vi "test Multi FPGA No Bitfile.vi"(8 "error in (no error)":errorcluster, 11 "TestCase in":refnum<class "Mutation Test Case.lvclass">) -> (0 "error out":errorcluster, 3 "TestCase out":refnum<class "Mutation Test Case.lvclass">)   [LabVIEW 2020, in "Mutation Test Case.lvclass"]
uses:
  Mutation Test Case.lvclass
  Shared/Properties.vi
  <vilib>/NI VeriStand/Custom Device API/Get Item Property (String).vi
  <vilib>/addons/_JKI Toolkits/VI Tester/TestCase.llb/TestCase.lvclass
  System Explorer/Engine Simulation Toolkit System Explorer.lvlib
  <vilib>/NI VeriStand/Custom Device API/Custom Device API.lvlib
  Shared/Engine Simulation Toolkit Shared.lvlib
  C:/Program Files (x86)/National Instruments/LabVIEW 2020/vi.lib/addons/_JKI Toolkits/VI Tester/TestCase.llb/TestCase.lvclass
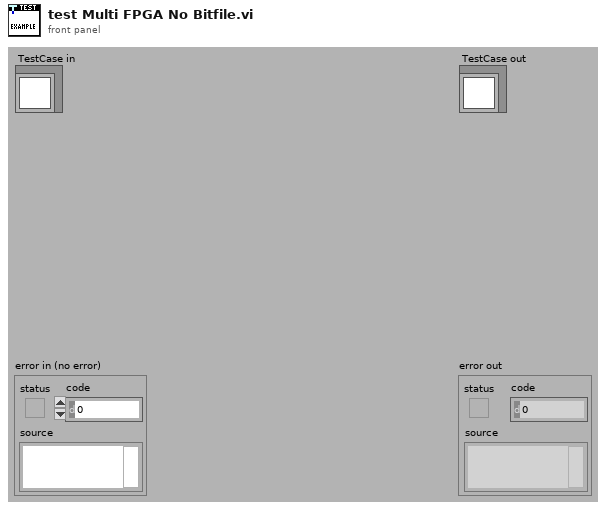
[diagram p1: front panel]
types:
  T1 = typedef "Custom Device API.lvlib/Custom Device Item Ref.ctl" = u64
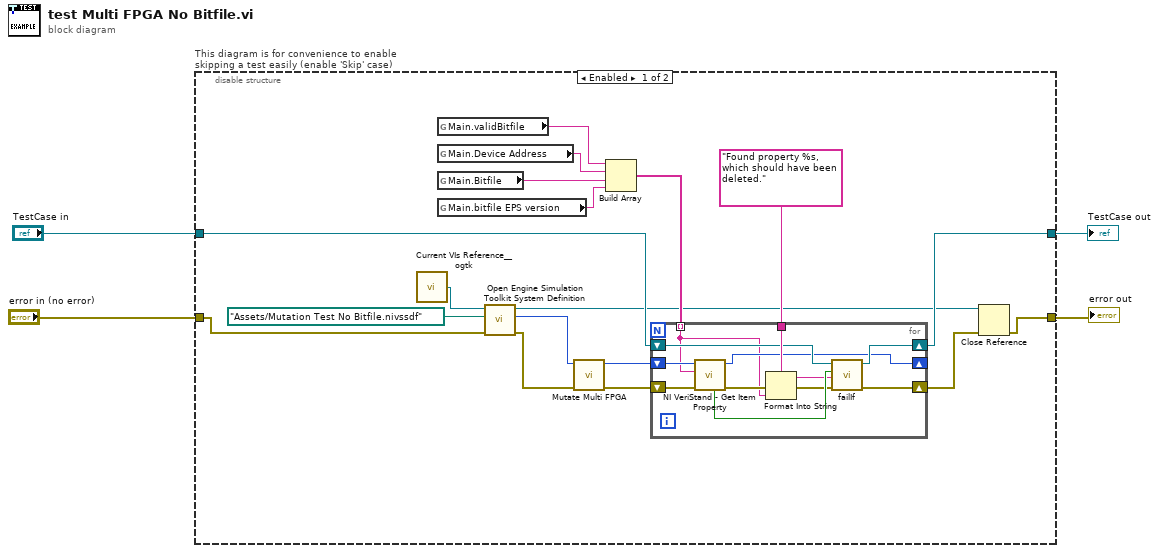
[diagram p0: block diagram]
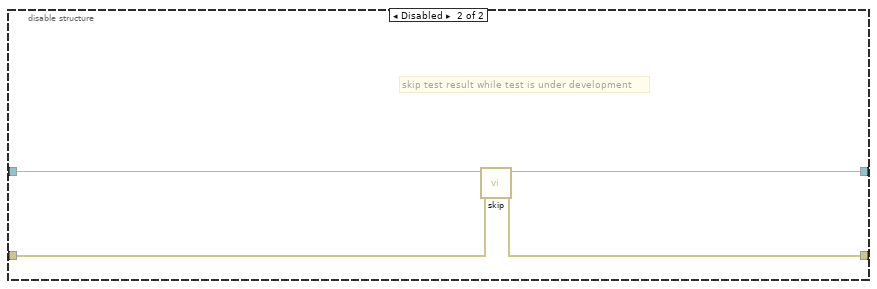
[diagram p2: hidden frame]
diagram:
  n1 = disable-structure "This diagram is for convenience to enable skipping a test easily (enable 'Skip' case)" shown="Enabled" {
    disable-tunnel: "TestCase in" -> [w16 w38]
    disable-tunnel: [w8 w36] -> w1
    disable-tunnel: [w6 w37] -> w3
    disable-tunnel: "error in (no error)" -> [w20 w35]
    frame Enabled {
      n2 = call <userlib>:"Current VIs Reference__ogtk.vi"() -> ("Current VI's reference"=w22:refnum<vi>)  [unwired: 5 in]
      n3 = global read "Properties.vi" "Main.validBitfile"() -> (w14:string)
      n4 = global read "Properties.vi" "Main.Device Address"() -> (w15:string)
      n5 = global read "Properties.vi" "Main.Bitfile"() -> (w13:string)
      n6 = global read "Properties.vi" "Main.bitfile EPS version"() -> (w12:string)
      n7 = call "Open Engine Simulation Toolkit System Definition.vi"("error in (no error)"=w20, "System Definition Path"=path "Assets/Mutation Test No Bitfile.nivssdf" ("Absolute or Relative Path"), "Current VI in"=w22) -> ("error out"=w7:errorcluster, "Engine Simulation Toolkit NodeID"=w19:u64, "SystemDefinition"=w5:refnum<k24>)  [unwired: 6 in]
      n8 = call "Mutate Multi FPGA.vi"("error in (no error)"=w7, "Device Ref in"=w19) -> ("error out"=w17:errorcluster, "Device Ref out"=w18:T1)  [unwired: 8 in]
      n9 = Build Array(w14, w15, w13, w12) -> (w11:string[])
      n10 = for {
        shift-right: [w30] -> w9
        shift-left: w17 -> [w33]
        shift-right: [w31] -> w8
        shift-left: w16 -> [w28]
        tunnel: w11 -> [w23] mode=indexing
        tunnel: "Found property %s, which should have been deleted." ("format string") -> [w29]
        shift-right: [w24] -> _
        shift-left: w18 -> [w34]
        n11 = call-poly <vilib>:"NI VeriStand - Get Item Property.vi"("error in (no error)"=w33, "Property Name"=w23, "Item Ref in"=w34) -> ("error out"=w27:errorcluster, "Item Ref out"=w24:T1, "Found?"=w32:bool)  [unwired: 5 in, 1 out]
        n12 = Format Into String(format string=w29, error in=w27, w23) -> (resulting string=w25:string, error out=w26:errorcluster)  [unwired: 1 in]
        n13 = call-dynamic "failIf.vi"("error in (no error)"=w26, "message (\"\")"=w25, "fail"=w32, "TestCase in"=w28) -> ("error out"=w30:errorcluster, "TestCase out"=w31:refnum<class "Mutation Test Case.lvclass">)  [unwired: 6 in]
      }
      n14 = Close Reference(reference=w5, error in (no error)=w9) -> (error out=w6:errorcluster)
    }
    frame Disabled {
      # "skip test result while test is under development"
      n15 = call <vilib>:"skip.vi"("error in (no error)"=w35, "TestCase in"=w38) -> ("error out"=w37:errorcluster, "TestCase out"=w36:refnum<class "Mutation Test Case.lvclass">)  [unwired: 8 in]
    }
  }
  "error out" <- w3
  "TestCase out" <- w1
